vi "MathCad_Easy_Numeric_Set_Multiple_Var.vi"(8 "error in (no error)":errorcluster, 9 "Data In":T2(array[cluster]) {"value" format="%.2f"}, 11 "Mathcad Reference":T1) -> (0 "error out":errorcluster, 3 "Mathcad Reference":T1)   [LabVIEW 2015]
doc: "Sets numeric values in Mathcad. You can also use this VI to reset a variable that has already been set once. It is only dependent upon the variable name. The variables won't appear in the Mathcad worksheet, but are defined at the very beginning of the worksheet.\n\nInputs \n Wrksht Ref--ActiveX Reference to Mathcad Worksheet Class\n Data In-- Names and Data for the Variable to set.\n Array of Clusters\n Cluster (2 elements)\n Value (Double)\n New Variable Name(String)\nOutputs \n Wrksht Ref--ActiveX Reference to Mathcad Worksheet Class"
uses:
  Mathcad Reference.ctl
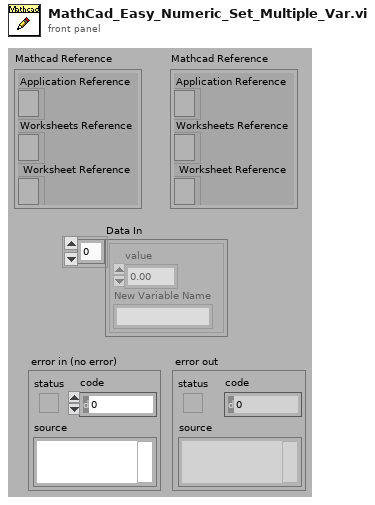
[diagram p1: front panel]
types:
  T1 = typedef "Mathcad Reference.ctl" = cluster{"Application Reference":refnum<k7>, "Worksheets Reference":refnum<k7>, " Worksheet Reference":refnum<k7>}
  T2 = cluster{"value":dbl, "New Variable Name":string}[]
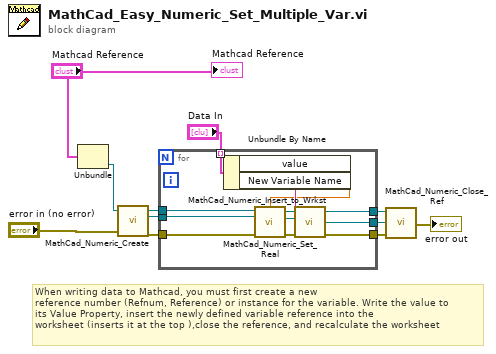
[diagram p0: block diagram]
diagram:
  # "When writing data to Mathcad, you must first create a new \nreference number (Refnum, Reference) or instance for the variable. Write the value to\nits Value Property, insert the newly defined variable reference into the\nworksheet (inserts it at the top ),close the reference, and recalculate the worksheet"
  n1 = Unbundle("Mathcad Reference") -> ("Worksheet Reference"=w4:refnum<k7>)  [unwired: 2 out]
  n2 = call "MathCad_Numeric_Create.vi"("error in (no error)"="error in (no error)", "Worksheet Reference In"=w4) -> ("error out"=w8:errorcluster, "Mathcad.INumericValue Reference Out"=w9:refnum<k7>, "Worksheet Reference Out"=w10:refnum<k7>)  [unwired: 1 in]
  n3 = for {
    tunnel: "Data In" -> [w20] mode=indexing
    tunnel: [w18] -> w6
    tunnel: [w17] -> w7
    tunnel: [w16] -> w1
    tunnel: w8 -> [w15]
    tunnel: w9 -> [w14]
    tunnel: w10 -> [w13]
    n4 = Unbundle By Name(w20) -> ("value"=w12:dbl, "New Variable Name"=w19:string)
    n5 = call "MathCad_Numeric_Set_Real.vi"("Worksheet Reference In"=w13, "Real"=w12, "Mathcad.INumericValue Refnum In"=w14, "error in"=w15) -> ("Worksheet Reference Out"=w23:refnum<k7>, "Mathcad.INumericValue Refnum Out"=w22:refnum<k7>, "error out"=w21:errorcluster)  [unwired: 9 in]
    n6 = call "MathCad_Numeric_Insert_to_Wrkst.vi"("error out 2"=w21, "New Variable Name"=w19, "Mathcad.INumericValue Ref In"=w22, "Wrksht Ref In"=w23) -> ("error out"=w16:errorcluster, "Mathcad.INumericValue Ref Out"=w17:refnum<k7>, "Wrksht Ref Out"=w18:refnum<k7>)
  }
  n7 = call "MathCad_Numeric_Close_Ref.vi"("error in"=w1, "Mathcad.INumericValue Reference"=w7, "IMathcadWorksheet Reference"=w6) -> ("error out"=→"error out":errorcluster)  [unwired: 2 in, 1 out]
  "Mathcad Reference" <- "Mathcad Reference"
